vi "DialogExamples.vi"() -> ()   [LabVIEW 2018, in "LcWebView.lvclass"]
uses:
  LcWebView.lvclass
panel:
  out "Error Out":errorcluster
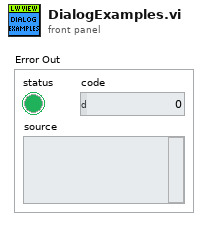
[diagram p1: front panel]
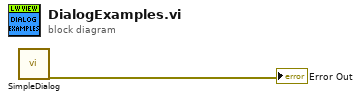
[diagram p0: block diagram]
diagram:
  n1 = call "SimpleDialog.vi"() -> ("error out"=→"Error Out":errorcluster)  [unwired: 19 in]
